vi "Initialise.vi"(8 "error in (no error)":errorcluster, 10 "Message in":refnum<class "InitialiseMessage.lvclass">, 11 "Autofocus in":refnum<class "Autofocus.lvclass">) -> (0 "error out":errorcluster, 3 "Autofocus out":refnum<class "Autofocus.lvclass">)   [LabVIEW 2012, in "Autofocus.lvclass"]
doc: "This method is called when an initialise message is received. It mainly initialises the RabbitMQ connectivity. \n\nOverride this method when your component needs special initialisation (e.g. of software or hardware resources). In that case, don't forget to call the parent for proper implementation. If your component owns subcomponents, they count as resources, so you have to initialise them by calling their own initialise functions"
uses:
  Autofocus.lvclass
  <vilib>/Distrio/Murmex/InitialiseMessage/InitialiseMessage.lvclass
  <vilib>/Distrio/Murmex/Murmex/Murmex.lvclass
  Autofocus.lvclass/Autofocus.ctl
panel:
  # "This method is called when the INTIALISE\ntrigger is sent. \n\nOverride this method when your component needs to\nrespond to this trigger. \n\nCall parent for proper implementation"
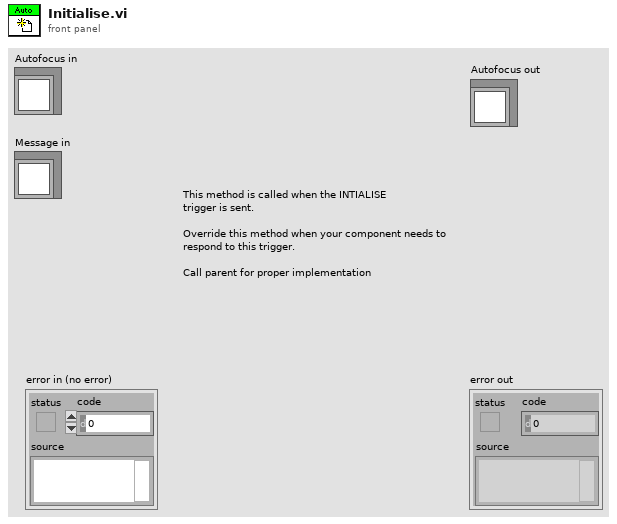
[diagram p1: front panel]
types:
  T1 = typedef "Autofocus.lvclass/number of subregions.ctl" = i32
  T2 = typedef "Image Type" = u32
  T3 = typedef "IMAQ Image.ctl" = refnum<image>
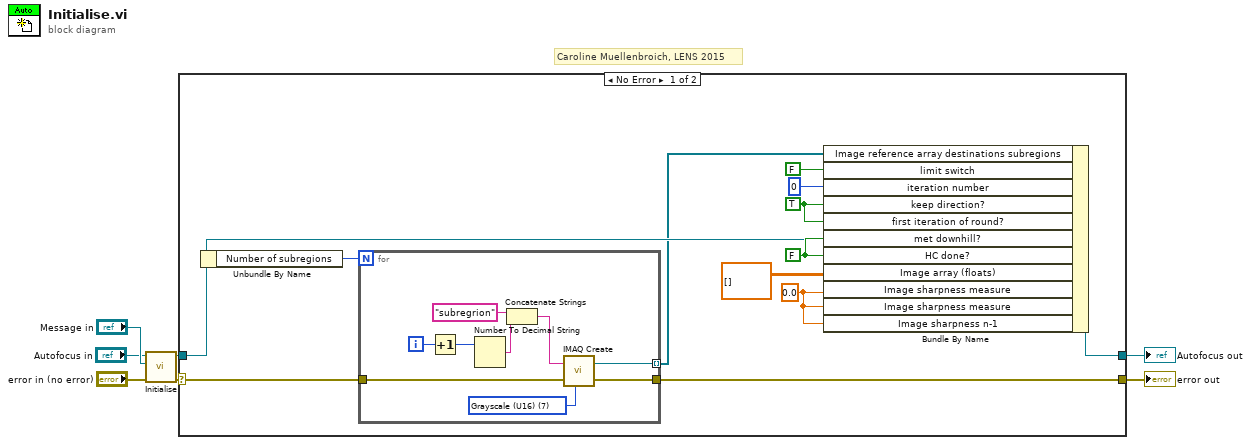
[diagram p0: block diagram]
diagram:
  # "Caroline Muellenbroich, LENS 2015"
  n1 = call-parent "Initialise.vi"("error in (no error)"="error in (no error)", "Message in"="Message in", "Murmex in"="Autofocus in") -> ("error out"=w4:errorcluster, "Murmex out"=w2:refnum<class "Autofocus.lvclass">)  [unwired: 7 in]
  n2 = case shown="No Error" w4 {
    selector: w4 -> [w11 w29]
    tunnel: [w10 w29] -> w3
    tunnel: w2 -> [w9 w30]
    tunnel: [w19 w30] -> w1
    frame No Error {
      w16 = TRUE ("Runtime cluster.keep direction?")
      w15 = FALSE ("Runtime cluster.done?")
      w17 = 0.0 ("Runtime cluster.Image sharpness measure")
      n3 = Unbundle By Name(w9) -> ("Number of subregions"=w12:T1)
      n4 = for {
        N: w12 -> [_]
        tunnel: w11 -> [w23]
        tunnel: [w22] -> w10
        tunnel: [w20] -> w8 mode=indexing
        i -> [w28]
        w21 = T2 7 items=["Grayscale (U8)", "Grayscale (I16)", "Grayscale (SGL)", "Complex (CSG)", "RGB (U32)", "HSL (U32)", "RGB (U64)", "Grayscale (U16)"] ("Image Type")
        n5 = Increment(x=w28) -> (x+1=w26:i32)
        n6 = Number To Decimal String(number=w26) -> (decimal integer string=w25:string)  [unwired: 1 in]
        n7 = Concatenate Strings("subregrion" ("string"), w25) -> (w27:string)
        n8 = call "IMAQ Create"("Image Name"=w27, "Image Type"=w21, "error in (no error)"=w23) -> ("New Image"=w20:T3, "error out"=w22:errorcluster)  [unwired: 2 in]
      }
      n9 = Bundle By Name(cluster=w9, "Image reference array destinations subregions"=w8, "limit switch"=FALSE ("Runtime cluster.limit switch"), "iteration number"=0 ("Runtime cluster.iteration number"), "keep direction?"=w16, "first iteration of round?"=w16, "met downhill?"=w15, "HC done?"=w15, "Image array (floats)"=sgl[][] [] ("Runtime cluster.Image array (floats)"), "Image sharpness measure"=w17, "Image sharpness measure"=w17, "Image sharpness n-1"=w17) -> (w19:refnum<class "Autofocus.lvclass">)
    }
    frame Error {
    }
  }
  "error out" <- w3
  "Autofocus out" <- w1
